vi "clicks.vi"(11 "reset":bool) -> (3 "function return":i32)   [LabVIEW 2017, in "HapticSTM.lvlib"]
doc: "extern \"C\" __declspec(dllexport) int clicks(bool reset);"
uses:
  <userlib>/HapticSTM/Feedbackless - Testdata/Zthreshholdtesting Folder/HapticSTM.lvlib
  <userlib>/HapticSTM/HapticSTM.dll
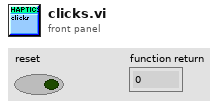
[diagram p1: front panel]
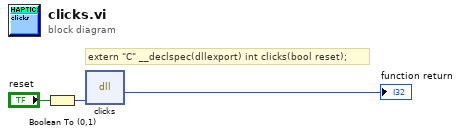
[diagram p0: block diagram]
diagram:
  # "extern \"C\" __declspec(dllexport) int clicks(bool reset);"
  n1 = Boolean To (0,1)(Boolean="reset") -> (0, 1=w1:i16)
  n2 = dll-call lib="C:/Program Files/National Instruments/LabVIEW 2019/user.lib/HapticSTM/HapticSTM.*" fn="clicks"("reset"=w1) -> (→"function return":i32)  [unwired: 4 in, 2 out]
